vi "SPCM_count_GPIB.vi"(11 "SR400 GPIB Address":string="23") -> (2 "Counts":dbl=5.0)   [LabVIEW 2015]
panel:
  out "time (s)":dbl=32.691
  out "Iteration":i32=44639252
  out "A_temp":dbl=18324.0
  # "On Windows/Linux, consider using the Instrument Driver Finder (Help>>Find Instrument Drivers) to search for an instrument driver for your instrument."
  # "1. Enter the GPIB address of the device.\n2. Choose the operation to perform (read, write, or both). \n3. Enter a timeout value in milliseconds.\n4. Enter the number of bytes to read.\n5. Type in the characters to be written to the instrument.\n6. Run the VI. \n\nIf you choose the \"Write then Read\" operation, the VI will write to the device first, then read from the device.\nBefore using this VI, you should consider initializing the bus with the \"GPIB Initialization\" function."
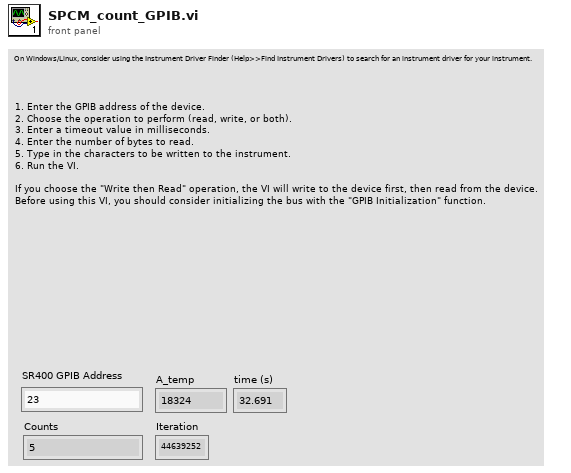
[diagram p1: front panel]
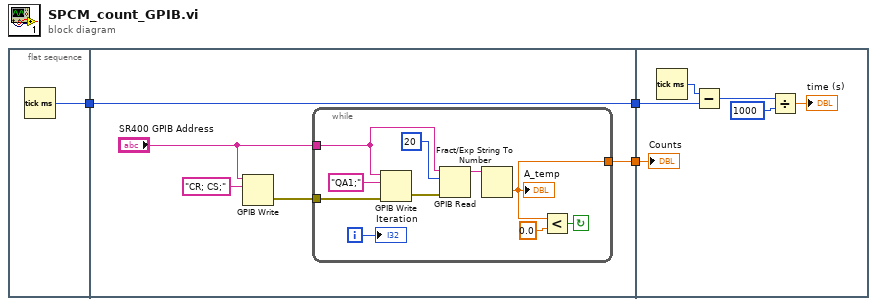
[diagram p0: block diagram]
diagram:
  n1 = flat-sequence {
    tunnel: [w4] -> w2
    tunnel: [w6] -> w3
    tunnel: w2 -> [w5]
    tunnel: [w5] -> w1
    tunnel: w3 -> [w25]
    tunnel: w1 -> [w20]
    frame #0 {
      n2 = Tick Count (ms)() -> (millisecond timer value=w4:u32)
    }
    frame #1 {
      n3 = GPIB Write(0:"SR400 GPIB Address", 1:"CR; CS;") -> (6:w7:errorcluster)  [unwired: 3 in, 1 out]
      n4 = while {
        tunnel: "SR400 GPIB Address" -> [w13]
        tunnel: w7 -> [w14]
        tunnel: [w11] -> w6
        i -> [w19]
        stop <- w10 continue-if-true
        n5 = GPIB Write(0:w13, 1:"QA1;" ("data string"), 3:w14) -> (6:w17:errorcluster)  [unwired: 2 in, 1 out]
        n6 = GPIB Read(0:w13, 1:20 ("byte count"), 3:w17) -> (5:w16:string)  [unwired: 2 in, 2 out]
        n7 = Fract/Exp String To Number(string=w16) -> (number=w11:dbl)  [unwired: 3 in, 1 out]
        "A_temp" <- w11
        n8 = Less?(x=w11, y=0.0) -> (x < y?=w10:bool)
        "Iteration" <- w19
      }
    }
    frame #2 {
      n9 = Tick Count (ms)() -> (millisecond timer value=w24:u32)
      n10 = Subtract(x=w24, y=w20) -> (x-y=w23:u32)
      n11 = Divide(x=w23, y=u32 1000) -> (x/y=→"time (s)":dbl)
      "Counts" <- w25
    }
  }
